vi "ADS1115.vi"() -> ()   [LabVIEW 2024]
uses:
  <vilib>/MakerHub/LINX/Private/Local IO/LinxI2cWrite.vi
  <vilib>/MakerHub/LINX/Public/Utilities/Check Channel.vi
  <vilib>/MakerHub/LINX/Private/Local IO/Handle Errors.vi
  <vilib>/MakerHub/LINX/Public/Utilities/Open Local.vi
  <vilib>/MakerHub/LINX/Private/Utilties/Generate Error.vi
  <vilib>/MakerHub/LINX/LMH-LINX.lvlib
panel:
  out "Channel 4":dbl format="%#.3f"
  in  "Channel 4":bool
  out "Channel 3":dbl format="%#.3f"
  in  "Channel 3":bool
  out "Channel 2":dbl format="%#.3f"
  in  "Channel 2":bool
  in  "Channel 1":bool
  in  "Conversion Mode":enum16{"One Channel", "Multiple Channel"}(ring)
  in  "Input Multiplexer (MUX)":u16(ring)=16384 items=["AIN0 - AIN1"=0, "AIN0 - AIN3"=4096, "AIN1 - AIN3"=8192, "AIN2 - AIN3"=12288, "AIN0 - GND"=16384, "AIN1 - GND"=20480, "AIN2 - GND"=24576, "AIN3 - GND"=28672]
  out "Channel 1":dbl format="%#.3f"
  out "Base Config":u16 format="%x"
  in  "Comparator Mode":u16(ring)=16 items=["Traditional"=0, "Window Comparator"=16]
  in  "Comparator Latch":u16(ring)=4 items=["Non-Latching"=0, "Latching"=4]
  in  "Comparator Polarity":u16(ring)=8 items=["Active Low"=0, "Active High"=8]
  in  "Comparator Queue":u16(ring)=3 items=["1 Conversion", "2 Conversions", "4 Conversions", "Disable Comparator"]
  in  "Data Rate":u16(ring)=224 items=["8 S/s"=0, "16 S/s"=32, "32 S/s"=64, "64 S/s"=96, "128 S/s"=128, "250 S/s"=160, "475 S/s"=192, "860 S/s"=224]
  in  "Mode Configuration":u16(ring) items=["Continuous Conversion"=0, "Single-Shot"=256]
  in  "Programmable Gain Amplifier (PGA)":u16(ring)=512 items=["±6.144 V"=0, "±4.096 V"=512, "±2.048 V"=1024, "±1.024 V"=1536, "±0.512 V"=2048, "±0.256 V"=2560, "±0.256 V"=3072, "±0.256 V"=3584]
  in  "Operational Status (OS)":u16(ring)=32768 items=["No Start"=0, "Start Conversion"=32768]
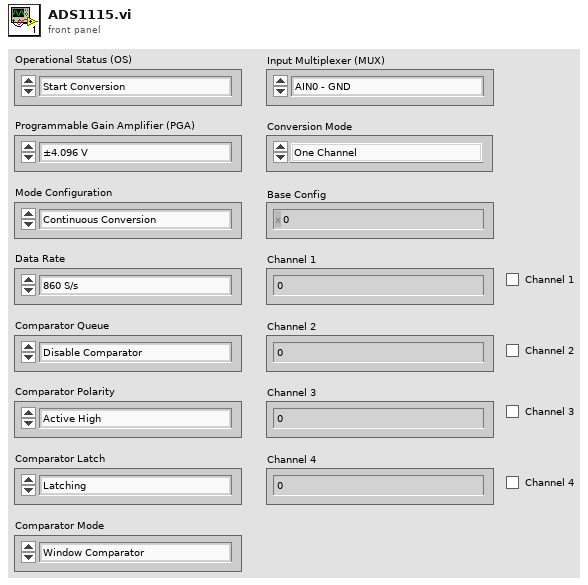
[diagram p1: front panel]
types:
  T1 = cluster{"I2C Slave Address":u8, "I2C Channel":u8}
  T2 = typedef "LMH-LINX.lvlib/LINX Ref.ctl" = cluster{"IO":T3, "Interface":T4, "LINX Device Config":T5}
  T3 = typedef "LMH-LINX.lvlib/Platform.ctl" = enum16{"Remote", "Local"}
  T4 = typedef "LMH-LINX.lvlib/Interface.ctl" = enum16{"Serial", "TCP"}
  T5 = typedef "LMH-LINX.lvlib/Device.lvlib/LINX Device Config.ctl" = cluster{"Interface":T4, "COM Port":refnum<visa-resource-name>, "TCP Configuration":T6, "Device Family":u8, "Device ID":u8, "Device Name":string, "TCP Ref":refnum<k5>, "Channels":T7}
  T6 = typedef "LMH-LINX.lvlib/Device.lvlib/TCP Config.ctl" = cluster{"IP Address":string, "Port":u16}
  T7 = typedef "LMH-LINX.lvlib/Channels.ctl" = cluster{"DI":u8[], "DO":u8[], "AI":u8[], "AO":u8[], "PWM":u8[], "QE":u8[], "UART":u8[], "I2C 2":u8[], "SPI":u8[], "CAN":u8[], "Servo":u8[], "AI Ref (V)":dbl, "AI Resolution (Bits)":u8, "AO Ref (V)":dbl, "AO Resolution (Bits)":u8}
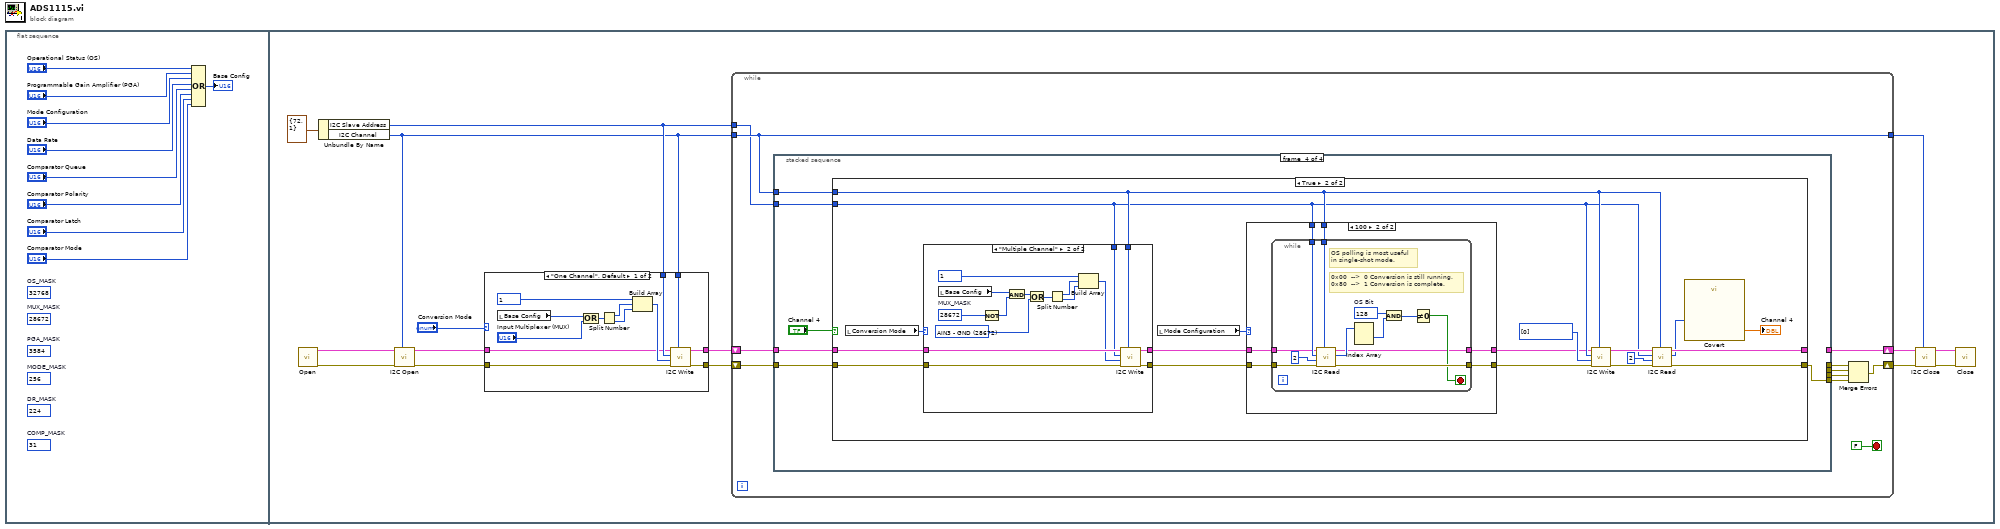
[diagram p0: block diagram]
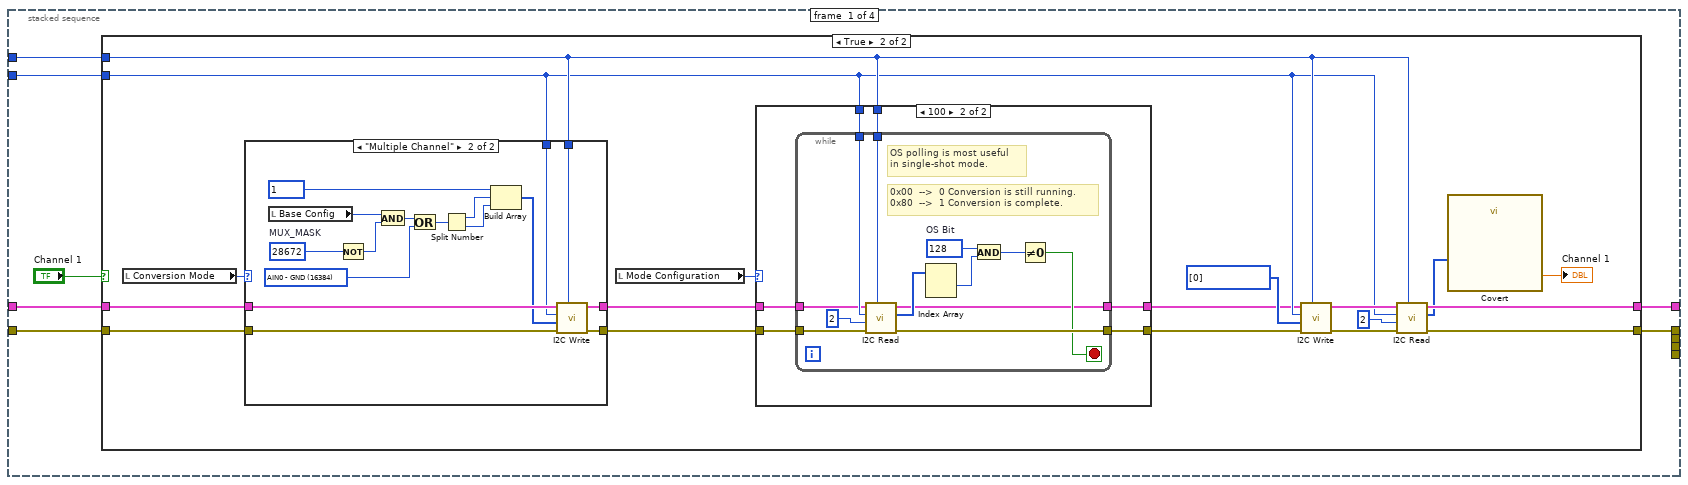
[diagram p3: hidden frame]
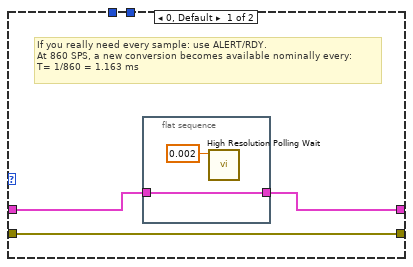
[diagram p5: hidden frame]
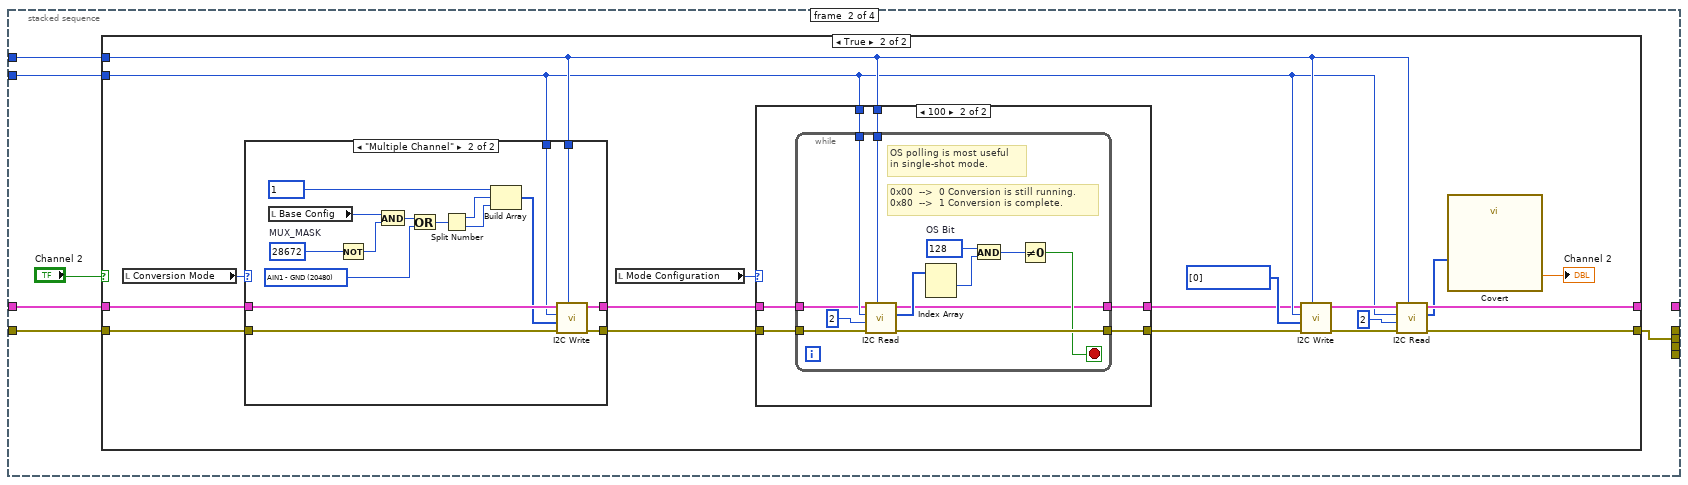
[diagram p7: hidden frame]
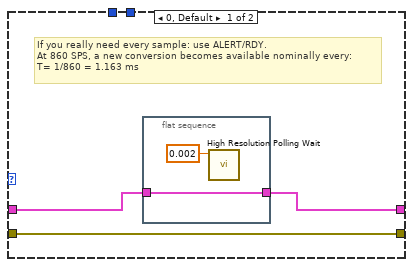
[diagram p9: hidden frame]
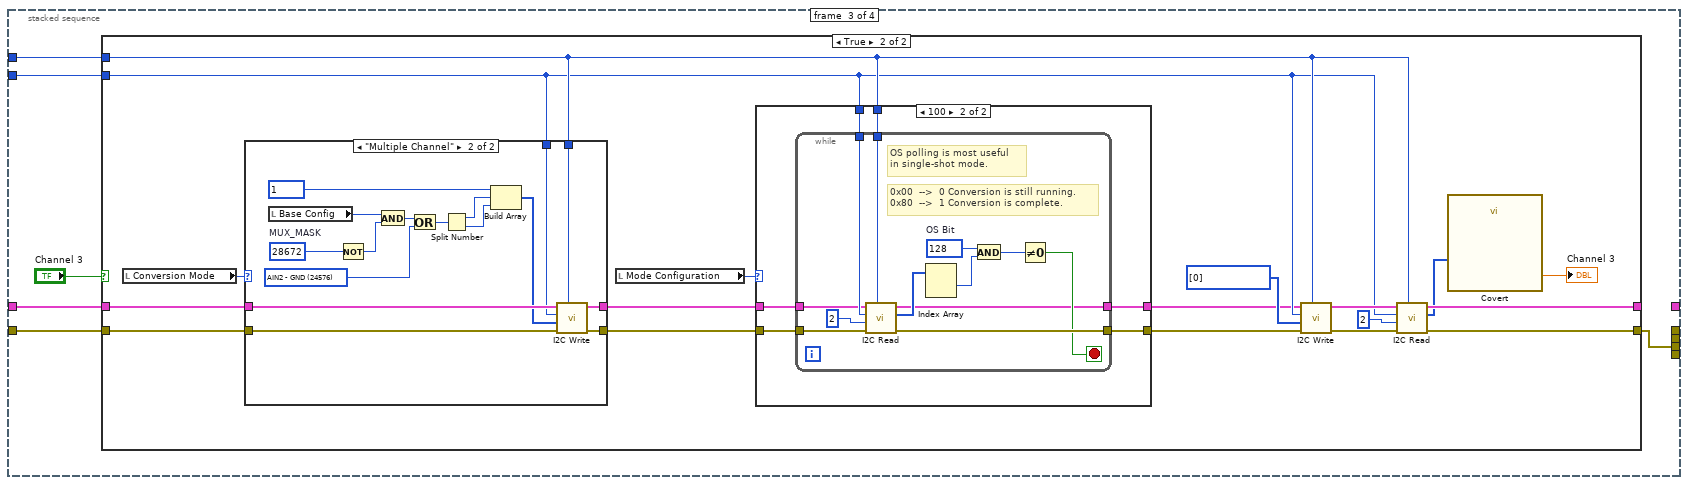
[diagram p11: hidden frame]
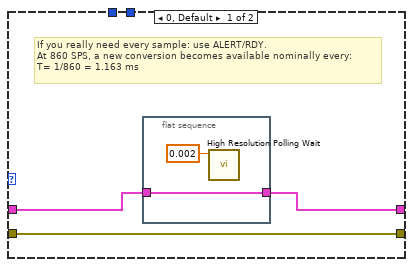
[diagram p13: hidden frame]
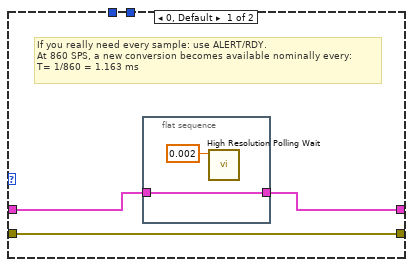
[diagram p16: hidden frame]
diagram:
  n1 = flat-sequence {
    frame #0 {
      (unwired) 31  # COMP_MASK
      (unwired) 224  # DR_MASK
      (unwired) 256  # MODE_MASK
      (unwired) 3584  # PGA_MASK
      (unwired) 28672  # MUX_MASK
      (unwired) 32768  # OS_MASK
      n2 = Compound Arithmetic op=OR("Operational Status (OS)", "Programmable Gain Amplifier (PGA)", "Mode Configuration", "Data Rate", "Comparator Queue", "Comparator Polarity", "Comparator Latch", "Comparator Mode") -> (→"Base Config":u16)
    }
    frame #1 {
      n3 = call-poly <vilib>:"Open.vi"() -> ("Error Out"=w15:errorcluster, "LINX Resource"=w23:T2)  [unwired: 9 in, 1 out]
      n4 = Unbundle By Name(T1 {"I2C Slave Address"=72, "I2C Channel"=1} ("Cluster")) -> ("I2C Slave Address"=w20:u8, "I2C Channel"=w11:u8)
      n5 = call <vilib>:"I2C Open.vi"("I2C Channel (0)"=w11, "Error In"=w15, "LINX Resource"=w23) -> ("Error Out"=w14:errorcluster, "LINX Resource"=w19:T2)  [unwired: 7 in]
      n6 = case shown="\"One Channel\", Default" "Conversion Mode" {
        tunnel: [w33 w38] -> w21
        tunnel: w20 -> [w32 _]
        tunnel: w19 -> [w31 w39]
        tunnel: w11 -> [w30 _]
        tunnel: w14 -> [w29 w38]
        tunnel: [w28 w39] -> w13
        frame "One Channel", Default {
          n7 = local read "Base Config"() -> (w37:u16)
          n8 = Compound Arithmetic op=OR(w37, "Input Multiplexer (MUX)") -> (w27:u16)
          n9 = Split Number(x=w27) -> (hi(x)=w26:u8, lo(x)=w25:u8)
          n10 = Build Array(1, w26, w25) -> (w35:i32[])
          n11 = call <vilib>:"I2C Write.vi"("I2C Channel"=w30, "Error In"=w29, "Data"=w35, "I2C Slave Address (0)"=w32, "LINX Resource"=w31) -> ("Error Out"=w33:errorcluster, "LINX Resource"=w28:T2)  [unwired: 5 in]
        }
        frame "Multiple Channel" {
        }
      }
      n12 = while {
        tunnel: w20 -> [w45]
        tunnel: w11 -> [w46]
        shift-right: [w50] -> w22
        shift-left: w13 -> [w49]
        shift-right: [w43] -> w17
        shift-left: w21 -> [w48]
        tunnel: [w46] -> w10
        stop <- FALSE stop-if-true
        n13 = stacked-sequence {
          tunnel: [w57 _ _ _] -> w50
          tunnel: w49 -> [w56 w124 w191 w258]
          tunnel: w48 -> [w55 w123 w190 w257]
          tunnel: [w54 _ _ _] -> w44
          tunnel: w46 -> [w53 w122 w189 w256]
          tunnel: w45 -> [w52 w121 w188 w255]
          tunnel: [_ w119 _ _] -> w42
          tunnel: [_ _ w186 _] -> w41
          tunnel: [_ _ _ w253] -> w40
          frame #0 {
            n14 = case shown="True" "Channel 1" {
              tunnel: [w59 w77] -> w57
              tunnel: w56 -> [w59 w69]
              tunnel: w55 -> [w58 w68]
              tunnel: [w58 w70] -> w54
              tunnel: w52 -> [_ w63]
              tunnel: w53 -> [_ w64]
              frame False {
              }
              frame True {
                n15 = local read "Conversion Mode"() -> (w67:enum16{"One Channel", "Multiple Channel"})
                n16 = case shown="\"Multiple Channel\"" w67 {
                  tunnel: [w102 w110] -> w62
                  tunnel: w69 -> [w102 w112]
                  tunnel: [w101 w109] -> w65
                  tunnel: w68 -> [w101 w111]
                  tunnel: w64 -> [_ w107]
                  tunnel: w63 -> [_ w106]
                  frame "One Channel", Default {
                  }
                  frame "Multiple Channel" {
                    w114 = u16 16384 items=["AIN0 - AIN1"=0, "AIN0 - AIN3"=4096, "AIN1 - AIN3"=8192, "AIN2 - AIN3"=12288, "AIN0 - GND"=16384, "AIN1 - GND"=20480, "AIN2 - GND"=24576, "AIN3 - GND"=28672] ("Input Multiplexer (MUX) 2")
                    w117 = u16 28672  # MUX_MASK
                    n17 = local read "Base Config"() -> (w118:u16)
                    n18 = Not(x=w117) -> (.not. x?=w116:u16)
                    n19 = And(x=w118, y=w116) -> (x .and. y?=w115:u16)
                    n20 = Or(x=w115, y=w114) -> (x .or. y?=w105:u16)
                    n21 = Split Number(x=w105) -> (hi(x)=w104:u8, lo(x)=w103:u8)
                    n22 = Build Array(1, w104, w103) -> (w108:i32[])
                    n23 = call <vilib>:"I2C Write.vi"("I2C Channel"=w107, "Error In"=w111, "Data"=w108, "I2C Slave Address (0)"=w106, "LINX Resource"=w112) -> ("Error Out"=w109:errorcluster, "LINX Resource"=w110:T2)  [unwired: 5 in]
                  }
                }
                n24 = local read "Mode Configuration"() -> (w60:u16)
                n25 = case shown="100" w60 {
                  tunnel: [w80 w88] -> w66
                  tunnel: w65 -> [w80 w87]
                  tunnel: w64 -> [_ w86]
                  tunnel: w63 -> [_ w85]
                  tunnel: w62 -> [w79 w84]
                  tunnel: [w78 w83] -> w61
                  frame 0, Default {
                    # "If you really need every sample: use ALERT/RDY.\nAt 860 SPS, a new conversion becomes available nominally every:\nT= 1/860 = 1.163 ms"
                    n26 = flat-sequence {
                      tunnel: w79 -> [w82]
                      tunnel: [w82] -> w78
                      frame #0 {
                        n27 = call <vilib>:"High Resolution Polling Wait.vi"("seconds to wait"=0.002) -> ()  [unwired: 10 in, 1 out]
                      }
                    }
                  }
                  frame 100 {
                    n28 = while {
                      tunnel: [w99] -> w88
                      tunnel: w87 -> [w89]
                      tunnel: w86 -> [w93]
                      tunnel: w85 -> [w92]
                      tunnel: w84 -> [w90]
                      tunnel: [w91] -> w83
                      stop <- w94 stop-if-true
                      w97 = 128  # OS Bit
                      # "0x00  -->  0\tConversion is still running.\n0x80  -->  1\tConversion is complete."
                      # "OS polling is most useful \nin single-shot mode."
                      n29 = call <vilib>:"I2C Read.vi"("I2C Channel"=w93, "Error In"=w89, "Bytes To Read"=u8 2, "I2C Slave Address (0)"=w92, "LINX Resource"=w90) -> ("Error Out"=w99:errorcluster, "Data"=w98:u8[], "LINX Resource"=w91:T2)  [unwired: 4 in]
                      n30 = Index Array(array=w98) -> (element #1=w96:u8)  [unwired: 2 in, 1 out]
                      n31 = And(x=w97, y=w96) -> (x .and. y?=w95:i32)
                      n32 = Not Equal To 0?(x=w95) -> (x != 0?=w94:bool)
                    }
                  }
                }
                n33 = call <vilib>:"I2C Write.vi"("I2C Channel"=w64, "Error In"=w66, "Data"=i32[] [0], "I2C Slave Address (0)"=w63, "LINX Resource"=w61) -> ("Error Out"=w75:errorcluster, "LINX Resource"=w71:T2)  [unwired: 5 in]
                n34 = call <vilib>:"I2C Read.vi"("I2C Channel"=w64, "Error In"=w75, "Bytes To Read"=u8 2, "I2C Slave Address (0)"=w63, "LINX Resource"=w71) -> ("Error Out"=w70:errorcluster, "Data"=w73:u8[], "LINX Resource"=w77:T2)  [unwired: 4 in]
                n35 = call "Covert.vi"("Data"=w73) -> ("Value"=→"Channel 1":dbl)  [unwired: 10 in]
              }
            }
          }
          frame #1 {
            n36 = case shown="True" "Channel 2" {
              tunnel: [w126 w144] -> _
              tunnel: w124 -> [w126 w137]
              tunnel: w123 -> [w125 w136]
              tunnel: [w125 w138] -> w119
              tunnel: w121 -> [_ w131]
              tunnel: w122 -> [_ w132]
              frame False {
              }
              frame True {
                n37 = local read "Conversion Mode"() -> (w135:enum16{"One Channel", "Multiple Channel"})
                n38 = case shown="\"Multiple Channel\"" w135 {
                  tunnel: [w169 w177] -> w130
                  tunnel: w137 -> [w169 w179]
                  tunnel: [w168 w176] -> w133
                  tunnel: w136 -> [w168 w178]
                  tunnel: w132 -> [_ w174]
                  tunnel: w131 -> [_ w173]
                  frame "One Channel", Default {
                  }
                  frame "Multiple Channel" {
                    w181 = u16 20480 items=["AIN0 - AIN1"=0, "AIN0 - AIN3"=4096, "AIN1 - AIN3"=8192, "AIN2 - AIN3"=12288, "AIN0 - GND"=16384, "AIN1 - GND"=20480, "AIN2 - GND"=24576, "AIN3 - GND"=28672] ("Input Multiplexer (MUX) 2")
                    w184 = u16 28672  # MUX_MASK
                    n39 = local read "Base Config"() -> (w185:u16)
                    n40 = Not(x=w184) -> (.not. x?=w183:u16)
                    n41 = And(x=w185, y=w183) -> (x .and. y?=w182:u16)
                    n42 = Or(x=w182, y=w181) -> (x .or. y?=w172:u16)
                    n43 = Split Number(x=w172) -> (hi(x)=w171:u8, lo(x)=w170:u8)
                    n44 = Build Array(1, w171, w170) -> (w175:i32[])
                    n45 = call <vilib>:"I2C Write.vi"("I2C Channel"=w174, "Error In"=w178, "Data"=w175, "I2C Slave Address (0)"=w173, "LINX Resource"=w179) -> ("Error Out"=w176:errorcluster, "LINX Resource"=w177:T2)  [unwired: 5 in]
                  }
                }
                n46 = local read "Mode Configuration"() -> (w128:u16)
                n47 = case shown="100" w128 {
                  tunnel: [w147 w155] -> w134
                  tunnel: w133 -> [w147 w154]
                  tunnel: w132 -> [_ w153]
                  tunnel: w131 -> [_ w152]
                  tunnel: w130 -> [w146 w151]
                  tunnel: [w145 w150] -> w129
                  frame 0, Default {
                    # "If you really need every sample: use ALERT/RDY.\nAt 860 SPS, a new conversion becomes available nominally every:\nT= 1/860 = 1.163 ms"
                    n48 = flat-sequence {
                      tunnel: w146 -> [w149]
                      tunnel: [w149] -> w145
                      frame #0 {
                        n49 = call <vilib>:"High Resolution Polling Wait.vi"("seconds to wait"=0.002) -> ()  [unwired: 10 in, 1 out]
                      }
                    }
                  }
                  frame 100 {
                    n50 = while {
                      tunnel: [w166] -> w155
                      tunnel: w154 -> [w156]
                      tunnel: w153 -> [w160]
                      tunnel: w152 -> [w159]
                      tunnel: w151 -> [w157]
                      tunnel: [w158] -> w150
                      stop <- w161 stop-if-true
                      w164 = 128  # OS Bit
                      # "0x00  -->  0\tConversion is still running.\n0x80  -->  1\tConversion is complete."
                      # "OS polling is most useful \nin single-shot mode."
                      n51 = call <vilib>:"I2C Read.vi"("I2C Channel"=w160, "Error In"=w156, "Bytes To Read"=u8 2, "I2C Slave Address (0)"=w159, "LINX Resource"=w157) -> ("Error Out"=w166:errorcluster, "Data"=w165:u8[], "LINX Resource"=w158:T2)  [unwired: 4 in]
                      n52 = Index Array(array=w165) -> (element #1=w163:u8)  [unwired: 2 in, 1 out]
                      n53 = And(x=w164, y=w163) -> (x .and. y?=w162:i32)
                      n54 = Not Equal To 0?(x=w162) -> (x != 0?=w161:bool)
                    }
                  }
                }
                n55 = call <vilib>:"I2C Write.vi"("I2C Channel"=w132, "Error In"=w134, "Data"=i32[] [0], "I2C Slave Address (0)"=w131, "LINX Resource"=w129) -> ("Error Out"=w142:errorcluster, "LINX Resource"=w139:T2)  [unwired: 5 in]
                n56 = call <vilib>:"I2C Read.vi"("I2C Channel"=w132, "Error In"=w142, "Bytes To Read"=u8 2, "I2C Slave Address (0)"=w131, "LINX Resource"=w139) -> ("Error Out"=w138:errorcluster, "Data"=w140:u8[], "LINX Resource"=w144:T2)  [unwired: 4 in]
                n57 = call "Covert.vi"("Data"=w140) -> ("Value"=→"Channel 2":dbl)  [unwired: 10 in]
              }
            }
          }
          frame #2 {
            n58 = case shown="True" "Channel 3" {
              tunnel: [w193 w211] -> _
              tunnel: w191 -> [w193 w204]
              tunnel: w190 -> [w192 w203]
              tunnel: [w192 w205] -> w186
              tunnel: w188 -> [_ w198]
              tunnel: w189 -> [_ w199]
              frame False {
              }
              frame True {
                n59 = local read "Conversion Mode"() -> (w202:enum16{"One Channel", "Multiple Channel"})
                n60 = case shown="\"Multiple Channel\"" w202 {
                  tunnel: [w236 w244] -> w197
                  tunnel: w204 -> [w236 w246]
                  tunnel: [w235 w243] -> w200
                  tunnel: w203 -> [w235 w245]
                  tunnel: w199 -> [_ w241]
                  tunnel: w198 -> [_ w240]
                  frame "One Channel", Default {
                  }
                  frame "Multiple Channel" {
                    w248 = u16 24576 items=["AIN0 - AIN1"=0, "AIN0 - AIN3"=4096, "AIN1 - AIN3"=8192, "AIN2 - AIN3"=12288, "AIN0 - GND"=16384, "AIN1 - GND"=20480, "AIN2 - GND"=24576, "AIN3 - GND"=28672] ("Input Multiplexer (MUX) 2")
                    w251 = u16 28672  # MUX_MASK
                    n61 = local read "Base Config"() -> (w252:u16)
                    n62 = Not(x=w251) -> (.not. x?=w250:u16)
                    n63 = And(x=w252, y=w250) -> (x .and. y?=w249:u16)
                    n64 = Or(x=w249, y=w248) -> (x .or. y?=w239:u16)
                    n65 = Split Number(x=w239) -> (hi(x)=w238:u8, lo(x)=w237:u8)
                    n66 = Build Array(1, w238, w237) -> (w242:i32[])
                    n67 = call <vilib>:"I2C Write.vi"("I2C Channel"=w241, "Error In"=w245, "Data"=w242, "I2C Slave Address (0)"=w240, "LINX Resource"=w246) -> ("Error Out"=w243:errorcluster, "LINX Resource"=w244:T2)  [unwired: 5 in]
                  }
                }
                n68 = local read "Mode Configuration"() -> (w195:u16)
                n69 = case shown="100" w195 {
                  tunnel: [w214 w222] -> w201
                  tunnel: w200 -> [w214 w221]
                  tunnel: w199 -> [_ w220]
                  tunnel: w198 -> [_ w219]
                  tunnel: w197 -> [w213 w218]
                  tunnel: [w212 w217] -> w196
                  frame 0, Default {
                    # "If you really need every sample: use ALERT/RDY.\nAt 860 SPS, a new conversion becomes available nominally every:\nT= 1/860 = 1.163 ms"
                    n70 = flat-sequence {
                      tunnel: w213 -> [w216]
                      tunnel: [w216] -> w212
                      frame #0 {
                        n71 = call <vilib>:"High Resolution Polling Wait.vi"("seconds to wait"=0.002) -> ()  [unwired: 10 in, 1 out]
                      }
                    }
                  }
                  frame 100 {
                    n72 = while {
                      tunnel: [w233] -> w222
                      tunnel: w221 -> [w223]
                      tunnel: w220 -> [w227]
                      tunnel: w219 -> [w226]
                      tunnel: w218 -> [w224]
                      tunnel: [w225] -> w217
                      stop <- w228 stop-if-true
                      w231 = 128  # OS Bit
                      # "0x00  -->  0\tConversion is still running.\n0x80  -->  1\tConversion is complete."
                      # "OS polling is most useful \nin single-shot mode."
                      n73 = call <vilib>:"I2C Read.vi"("I2C Channel"=w227, "Error In"=w223, "Bytes To Read"=u8 2, "I2C Slave Address (0)"=w226, "LINX Resource"=w224) -> ("Error Out"=w233:errorcluster, "Data"=w232:u8[], "LINX Resource"=w225:T2)  [unwired: 4 in]
                      n74 = Index Array(array=w232) -> (element #1=w230:u8)  [unwired: 2 in, 1 out]
                      n75 = And(x=w231, y=w230) -> (x .and. y?=w229:i32)
                      n76 = Not Equal To 0?(x=w229) -> (x != 0?=w228:bool)
                    }
                  }
                }
                n77 = call <vilib>:"I2C Write.vi"("I2C Channel"=w199, "Error In"=w201, "Data"=i32[] [0], "I2C Slave Address (0)"=w198, "LINX Resource"=w196) -> ("Error Out"=w209:errorcluster, "LINX Resource"=w206:T2)  [unwired: 5 in]
                n78 = call <vilib>:"I2C Read.vi"("I2C Channel"=w199, "Error In"=w209, "Bytes To Read"=u8 2, "I2C Slave Address (0)"=w198, "LINX Resource"=w206) -> ("Error Out"=w205:errorcluster, "Data"=w207:u8[], "LINX Resource"=w211:T2)  [unwired: 4 in]
                n79 = call "Covert.vi"("Data"=w207) -> ("Value"=→"Channel 3":dbl)  [unwired: 10 in]
              }
            }
          }
          frame #3 {
            n80 = case shown="True" "Channel 4" {
              tunnel: [w260 w278] -> _
              tunnel: w258 -> [w260 w271]
              tunnel: w257 -> [w259 w270]
              tunnel: [w259 w272] -> w253
              tunnel: w255 -> [_ w265]
              tunnel: w256 -> [_ w266]
              frame False {
              }
              frame True {
                n81 = local read "Conversion Mode"() -> (w269:enum16{"One Channel", "Multiple Channel"})
                n82 = case shown="\"Multiple Channel\"" w269 {
                  tunnel: [w303 w311] -> w264
                  tunnel: w271 -> [w303 w313]
                  tunnel: [w302 w310] -> w267
                  tunnel: w270 -> [w302 w312]
                  tunnel: w266 -> [_ w308]
                  tunnel: w265 -> [_ w307]
                  frame "One Channel", Default {
                  }
                  frame "Multiple Channel" {
                    w315 = u16 28672 items=["AIN0 - AIN1"=0, "AIN0 - AIN3"=4096, "AIN1 - AIN3"=8192, "AIN2 - AIN3"=12288, "AIN0 - GND"=16384, "AIN1 - GND"=20480, "AIN2 - GND"=24576, "AIN3 - GND"=28672] ("Input Multiplexer (MUX) 2")
                    w318 = u16 28672  # MUX_MASK
                    n83 = local read "Base Config"() -> (w319:u16)
                    n84 = Not(x=w318) -> (.not. x?=w317:u16)
                    n85 = And(x=w319, y=w317) -> (x .and. y?=w316:u16)
                    n86 = Or(x=w316, y=w315) -> (x .or. y?=w306:u16)
                    n87 = Split Number(x=w306) -> (hi(x)=w305:u8, lo(x)=w304:u8)
                    n88 = Build Array(1, w305, w304) -> (w309:i32[])
                    n89 = call <vilib>:"I2C Write.vi"("I2C Channel"=w308, "Error In"=w312, "Data"=w309, "I2C Slave Address (0)"=w307, "LINX Resource"=w313) -> ("Error Out"=w310:errorcluster, "LINX Resource"=w311:T2)  [unwired: 5 in]
                  }
                }
                n90 = local read "Mode Configuration"() -> (w262:u16)
                n91 = case shown="100" w262 {
                  tunnel: [w281 w289] -> w268
                  tunnel: w267 -> [w281 w288]
                  tunnel: w266 -> [_ w287]
                  tunnel: w265 -> [_ w286]
                  tunnel: w264 -> [w280 w285]
                  tunnel: [w279 w284] -> w263
                  frame 0, Default {
                    # "If you really need every sample: use ALERT/RDY.\nAt 860 SPS, a new conversion becomes available nominally every:\nT= 1/860 = 1.163 ms"
                    n92 = flat-sequence {
                      tunnel: w280 -> [w283]
                      tunnel: [w283] -> w279
                      frame #0 {
                        n93 = call <vilib>:"High Resolution Polling Wait.vi"("seconds to wait"=0.002) -> ()  [unwired: 10 in, 1 out]
                      }
                    }
                  }
                  frame 100 {
                    n94 = while {
                      tunnel: [w300] -> w289
                      tunnel: w288 -> [w290]
                      tunnel: w287 -> [w294]
                      tunnel: w286 -> [w293]
                      tunnel: w285 -> [w291]
                      tunnel: [w292] -> w284
                      stop <- w295 stop-if-true
                      w298 = 128  # OS Bit
                      # "0x00  -->  0\tConversion is still running.\n0x80  -->  1\tConversion is complete."
                      # "OS polling is most useful \nin single-shot mode."
                      n95 = call <vilib>:"I2C Read.vi"("I2C Channel"=w294, "Error In"=w290, "Bytes To Read"=u8 2, "I2C Slave Address (0)"=w293, "LINX Resource"=w291) -> ("Error Out"=w300:errorcluster, "Data"=w299:u8[], "LINX Resource"=w292:T2)  [unwired: 4 in]
                      n96 = Index Array(array=w299) -> (element #1=w297:u8)  [unwired: 2 in, 1 out]
                      n97 = And(x=w298, y=w297) -> (x .and. y?=w296:i32)
                      n98 = Not Equal To 0?(x=w296) -> (x != 0?=w295:bool)
                    }
                  }
                }
                n99 = call <vilib>:"I2C Write.vi"("I2C Channel"=w266, "Error In"=w268, "Data"=i32[] [0], "I2C Slave Address (0)"=w265, "LINX Resource"=w263) -> ("Error Out"=w276:errorcluster, "LINX Resource"=w273:T2)  [unwired: 5 in]
                n100 = call <vilib>:"I2C Read.vi"("I2C Channel"=w266, "Error In"=w276, "Bytes To Read"=u8 2, "I2C Slave Address (0)"=w265, "LINX Resource"=w273) -> ("Error Out"=w272:errorcluster, "Data"=w274:u8[], "LINX Resource"=w278:T2)  [unwired: 4 in]
                n101 = call "Covert.vi"("Data"=w274) -> ("Value"=→"Channel 4":dbl)  [unwired: 10 in]
              }
            }
          }
        }
        n102 = Merge Errors(w44, w42, w41, w40) -> (w43:errorcluster)
      }
      n103 = call <vilib>:"I2C Close.vi"("I2C Channel (0)"=w10, "Error In"=w17, "LINX Resource"=w22) -> ("Error Out"=w16:errorcluster, "LINX Resource"=w18:T2)  [unwired: 7 in]
      n104 = call <vilib>:"Close.vi"("Error In"=w16, "LINX Resource"=w18) -> ()  [unwired: 9 in, 1 out]
    }
  }
